vi "Subsystem_command_filter.vi"(10 "Subsystem name":string, 11 "Array of commands":string[](array[string])) -> (3 "Subsystem commands out":string[](array[string]))   [LabVIEW 2017, in "labview-standard-library.lvlib"]
uses:
  labview-standard-library.lvlib
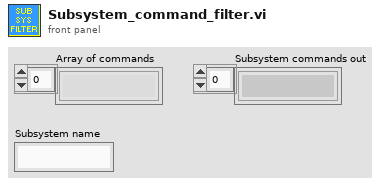
[diagram p1: front panel]
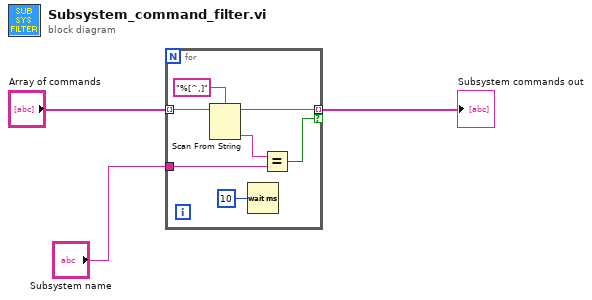
[diagram p0: block diagram]
diagram:
  n1 = for {
    tunnel: "Array of commands" -> [w9] mode=indexing
    tunnel: [w6] -> w2 mode=indexing if=w5
    tunnel: "Subsystem name" -> [w4]
    n2 = Scan From String(format string="%[^,]", input string=w9) -> (remaining string=w6:string, output 1=w7:string)  [unwired: 3 in, 2 out]
    n3 = Wait (ms)(milliseconds to wait=u32 10) -> ()  [unwired: 1 out]
    n4 = Equal?(x=w7, y=w4) -> (x = y?=w5:bool)
  }
  "Subsystem commands out" <- w2
